vi "VIrefParse.vi"(3 "Params":T1, 4 "VIA":string, 5 "String in":string) -> (2 "String out":string)   [LabVIEW 2012]
panel:
  out "Array 2":T2(array[cluster])
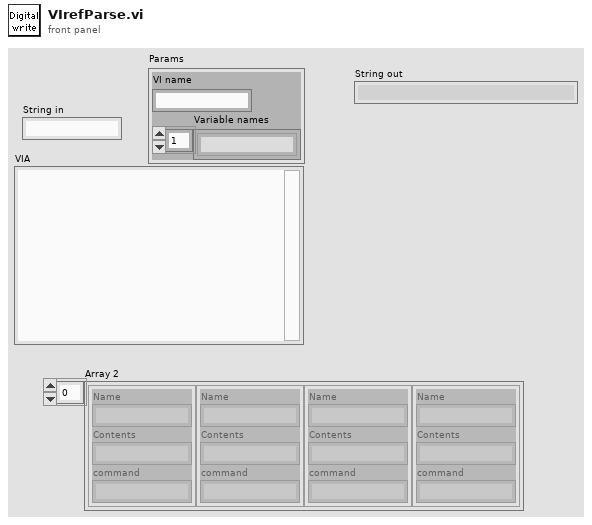
[diagram p1: front panel]
types:
  T1 = cluster{"VI name":string, "Variable names":string[]}
  T2 = cluster{"Name":string, "Contents":string, "command":string}[]
  T3 = cluster{"trimmed string":string, "Contents":string, "command":string}
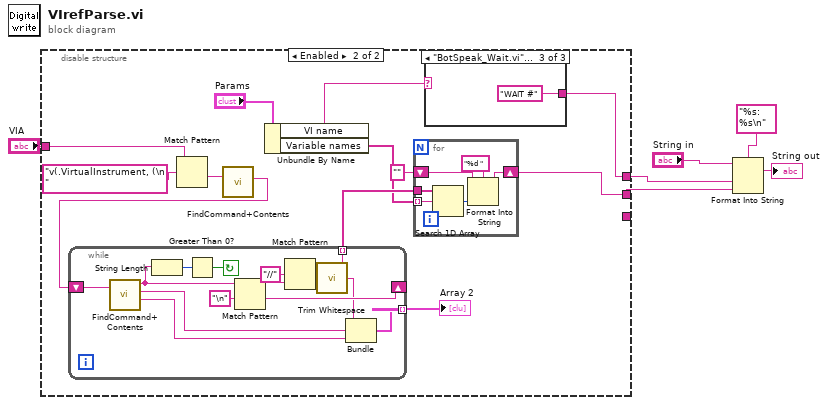
[diagram p0: block diagram]
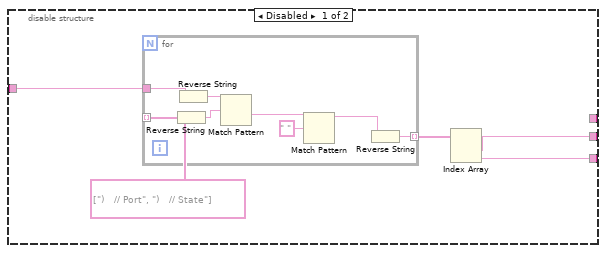
[diagram p2: hidden frame]
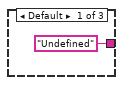
[diagram p3: hidden frame]
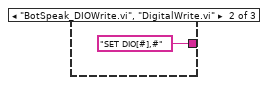
[diagram p4: hidden frame]
diagram:
  n1 = disable-structure shown="Enabled" {
    disable-tunnel: "VIA" -> [w11 w30]
    disable-tunnel: [w8 w22] -> w2
    disable-tunnel: [w7 _] -> _
    disable-tunnel: [_ w20] -> w1
    frame Disabled {
      n2 = for {
        tunnel: w11 -> [w19]
        tunnel: [w14] -> w9 mode=indexing
        tunnel: string[] [")   // Port", ")   // State"] -> [w12] mode=indexing
        n3 = Reverse String(1:w12) -> (0:w17:string)
        n4 = Reverse String(1:w19) -> (0:w18:string)
        n5 = Match Pattern(string=w18, regular expression=w17) -> (after substring=w15:string)  [unwired: 1 in, 3 out]
        n6 = Match Pattern(string=w15, regular expression=" ") -> (before substring=w13:string)  [unwired: 1 in, 3 out]
        n7 = Reverse String(1:w13) -> (0:w14:string)
      }
      n8 = Index Array(array=w9) -> (element #1=w8:string, element #2=w7:string)  [unwired: 2 in]
    }
    frame Enabled {
      n9 = Match Pattern(string=w30, regular expression="v(.VirtualInstrument, (\n   ") -> (after substring=w29:string)  [unwired: 1 in, 3 out]
      n10 = call "FindCommand+Contents.vi"("Via file in"=w29) -> ("Contents"=w27:string)  [unwired: 1 in, 3 out]
      n11 = while {
        shift-right: [w46] -> _
        shift-left: w27 -> [w53]
        tunnel: [w49] -> w28 mode=indexing
        tunnel: [w41] -> w26 mode=indexing
        stop <- w51 continue-if-true
        n12 = call "FindCommand+Contents.vi"("Via file in"=w53) -> ("left"=w45:string, "Contents"=w48:string, "command"=w50:string)  [unwired: 1 in, 1 out]
        n13 = String Length(string=w45) -> (length=w52:i32)
        n14 = Greater Than 0?(x=w52) -> (x > 0?=w51:bool)
        n15 = Match Pattern(string=w45, regular expression="\n") -> (before substring=w44:string, after substring=w46:string)  [unwired: 1 in, 2 out]
        n16 = Match Pattern(string=w44, regular expression="//") -> (after substring=w43:string)  [unwired: 1 in, 3 out]
        n17 = call <vilib>:"Trim Whitespace.vi"("string"=w43) -> ("trimmed string"=w41:string)  [unwired: 1 in]
        n18 = Bundle("trimmed string"=w41, "Contents"=w48, "command"=w50) -> (w49:T3)  [unwired: 1 in]
      }
      "Array 2" <- w28
      n19 = Unbundle By Name("Params") -> ("VI name"=w21:string, "Variable names"=w24:string[])
      n20 = for {
        tunnel: w24 -> [w40] mode=indexing
        tunnel: w26 -> [w38]
        shift-right: [w36] -> w22
        shift-left: "" -> [w35]
        n21 = Search 1D Array(1D array=w38, element=w40) -> (index of element=w39:i32)  [unwired: 1 in]
        n22 = Format Into String(format string="%d ", initial string=w35, w39) -> (resulting string=w36:string)  [unwired: 1 in, 1 out]
      }
      n23 = case shown="\"BotSpeak_Wait.vi\", \"VS_Wait.vi\"" w21 {
        tunnel: ["Undefined" ("format string") "SET DIO[#],#" ("format string") "WAIT #" ("format string")] -> w20
        frame Default {
        }
        frame "BotSpeak_DIOWrite.vi", "DigitalWrite.vi" {
        }
        frame "BotSpeak_Wait.vi", "VS_Wait.vi" {
        }
      }
    }
  }
  n24 = Format Into String(format string="%s: %s\n" ("regular expression"), initial string="String in", w1, w2) -> (resulting string=→"String out":string)  [unwired: 1 in, 1 out]
